vi "Find Item in ProjectItem.vi"(7 "Item Type":string, 8 "error in (no error)":errorcluster, 10 "Name":string, 11 "ProjectItem in":refnum<vi>) -> (0 "error out":errorcluster, 1 "Found ?":bool, 2 "Item Refnum out":refnum<vi>, 3 "ProjectItem out":refnum<vi>)   [LabVIEW 2019, in "gRPC Template Creation Utility.lvlib"]
uses:
  gRPC Template Creation Utility.lvlib
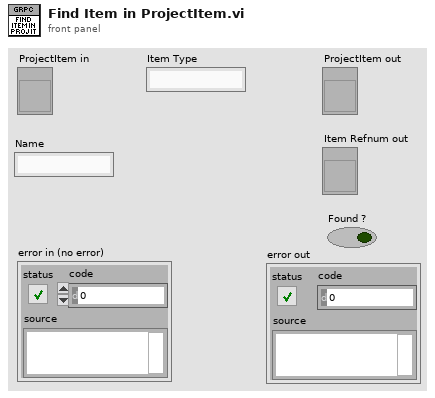
[diagram p1: front panel]
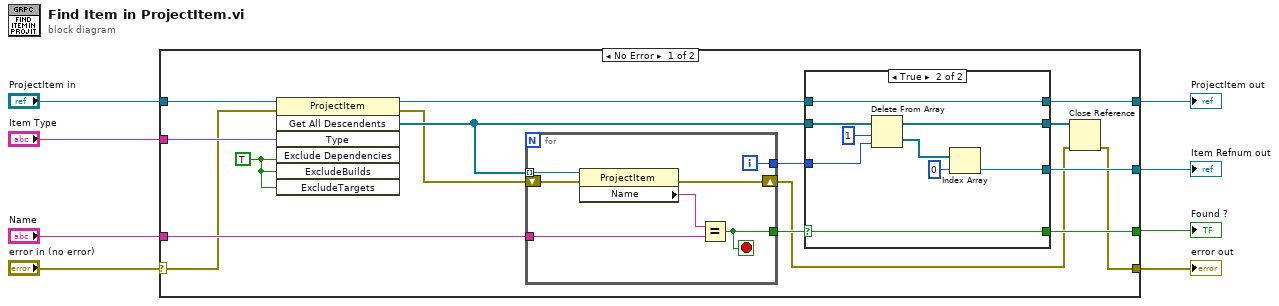
[diagram p0: block diagram]
diagram:
  n1 = case shown="No Error" "error in (no error)" {
    selector: "error in (no error)" -> [w18 w43]
    tunnel: "Name" -> [w24 _]
    tunnel: "Item Type" -> [w20 _]
    tunnel: "ProjectItem in" -> [w19 w44]
    tunnel: [w13 w44] -> w7
    tunnel: [w15 _] -> w5
    tunnel: [w17 _] -> w6
    tunnel: [w9 w43] -> w1
    frame No Error {
      w21 = TRUE ("ExcludeDependencies")
      n2 = invoke class="ProjectItem" method="Get All Descendents"(reference=w19, error in=w18, "Type"=w20, "Exclude Dependencies"=w21, "ExcludeBuilds"=w21, "ExcludeTargets"=w21) -> (reference out=w14:refnum<vi>, error out=w12:errorcluster, "All Descendents"=w22:refnum<vi>[])  [unwired: 1 in, 4 out]
      n3 = for {
        tunnel: w22 -> [w31] mode=indexing
        tunnel: [w29] -> w23
        tunnel: [w28] -> w16
        tunnel: w24 -> [w27]
        shift-right: [w25] -> w10
        shift-left: w12 -> [w26]
        i -> [w29]
        stop <- w28 stop-if-true
        n4 = property class="ProjectItem"(reference=w31, error in=w26) -> (error out=w25:errorcluster, "Name"=w30:string)  [unwired: 1 out]
        n5 = Equal?(x=w30, y=w27) -> (x = y?=w28:bool)
      }
      n6 = case shown="True" w16 {
        selector: w16 -> [_ w36]
        tunnel: w23 -> [_ w41]
        tunnel: w22 -> [w32 w40]
        tunnel: [_ w37] -> w17
        tunnel: [_ w36] -> w15
        tunnel: w14 -> [w33 w35]
        tunnel: [w33 w35] -> w13
        tunnel: [w32 w34] -> w11
        frame False {
        }
        frame True {
          n7 = Delete From Array(array=w40, length=1, index=w41) -> (deleted portion=w39:refnum<vi>[], array with subset deleted=w34:refnum<vi>[])
          n8 = Index Array(array=w39, index=0) -> (element=w37:refnum<vi>)
        }
      }
      n9 = Close Reference(reference=w11, error in (no error)=w10) -> (error out=w9:errorcluster)
    }
    frame Error {
    }
  }
  "ProjectItem out" <- w7
  "Item Refnum out" <- w6
  "Found ?" <- w5
  "error out" <- w1
